vi "PDCBMPSave.vi"(0 "DeviceNo":u32, 1 "FileName":string, 2 "Slide Refnum":refnum<vi>, 5 "ChildNo":u32, 11 "error in (no error)":errorcluster, 13 "File_Frame":cluster{"StartFrame":i32, "EndFrame":i32}) -> (15 "error out":errorcluster)   [LabVIEW 2015]
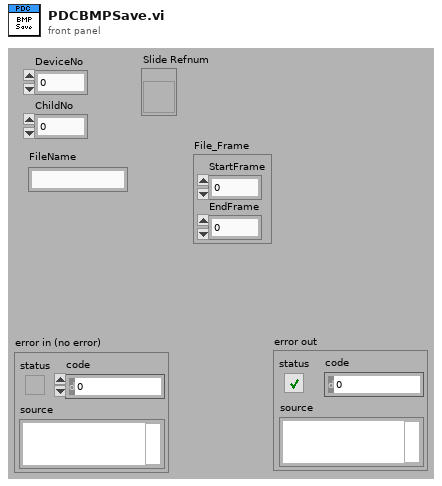
[diagram p1: front panel]
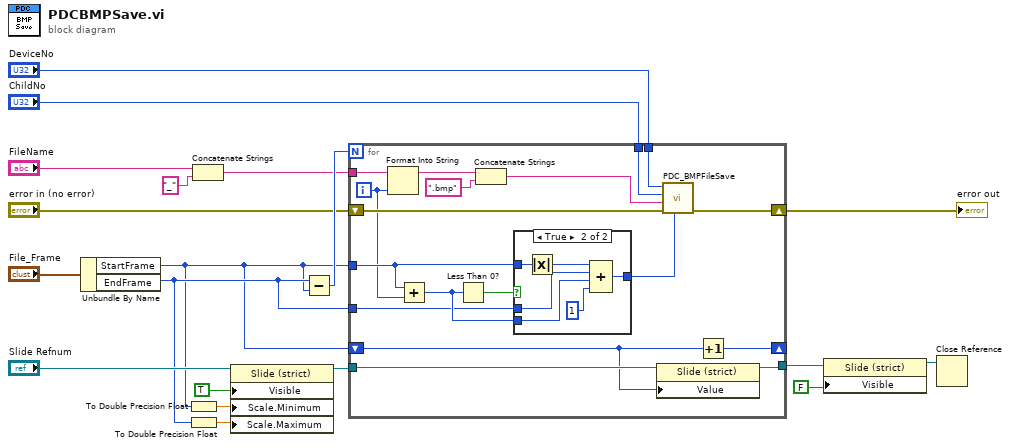
[diagram p0: block diagram]
diagram:
  n1 = Unbundle By Name("File_Frame") -> ("StartFrame"=w1:i32, "EndFrame"=w2:i32)
  n2 = To Double Precision Float(number=w1) -> (double precision float=w14:dbl)
  n3 = To Double Precision Float(number=w2) -> (double precision float=w15:dbl)
  n4 = Concatenate Strings("FileName", "_" ("string")) -> (w4:string)
  n5 = property class="Slide (strict)"(reference="Slide Refnum", "Visible"=TRUE ("表示"), "Scale.Minimum"=w14, "Scale.Maximum"=w15) -> (reference out=w8:refnum<vi>)  [unwired: 1 in, 1 out]
  n6 = Subtract(x=w2, y=w1) -> (x-y=w10:i32)
  n7 = for {
    N: w10 -> [_]
    tunnel: "DeviceNo" -> [w32]
    tunnel: "ChildNo" -> [w33]
    tunnel: w8 -> [w37]
    tunnel: [w36] -> w16
    shift-right: [w35] -> w6
    shift-left: "error in (no error)" -> [w34]
    tunnel: w4 -> [w31]
    tunnel: w1 -> [w25]
    tunnel: w2 -> [w23]
    shift-right: [w21] -> _
    shift-left: w1 -> [w20]
    i -> [w24]
    n8 = Format Into String(initial string=w31, w24) -> (resulting string=w29:string)  [unwired: 2 in, 1 out]
    n9 = Add(x=w25, y=w24) -> (x+y=w26:i32)
    n10 = Less Than 0?(x=w26) -> (x < 0?=w27:bool)
    n11 = Concatenate Strings(w29, ".bmp" ("string")) -> (w28:string)
    n12 = case shown="True" w27 {
      tunnel: w26 -> [w38 w41]
      tunnel: [w38 w39] -> w22
      tunnel: w23 -> [_ w42]
      tunnel: w25 -> [_ w44]
      frame False {
      }
      frame True {
        n13 = Absolute Value(x=w44) -> (abs(x)=w43:i32)
        n14 = Compound Arithmetic op=ADD(w43, w42, w41, 1 ("値")) -> (w39:i32)
      }
    }
    n15 = property class="Slide (strict)"(reference=w37, "Value"=w20) -> (reference out=w36:refnum<vi>)  [unwired: 1 in, 1 out]
    n16 = call "PDC_BMPFileSave.vi"("FrameNo"=w22, "error in (no error)"=w34, "FileName"=w28, "ChildNo"=w33, "DeviceNo"=w32) -> ("error out"=w35:errorcluster)  [unwired: 4 in, 2 out]
    n17 = Increment(x=w20) -> (x+1=w21:i32)
  }
  "error out" <- w6
  n18 = property class="Slide (strict)"(reference=w16, "Visible"=FALSE ("表示")) -> (reference out=w18:refnum<vi>)  [unwired: 1 in, 1 out]
  n19 = Close Reference(reference=w18) -> ()  [unwired: 1 in, 1 out]
